vi "Host - 2954 - 6592R Rx Streaming.vi"() -> ()   [LabVIEW 2018, in "Stream-2954-6592R.lvlib"]
uses:
  Stream-2954-6592R.lvlib
  <vilib>/userDefined/Silver/nirio_resource_slv.ctl
  TypeDefs/USRP Configuration.ctl
  TypeDefs/Rx Config.ctl
  2954/SubVIs/Start Trigger.ctl
  TDMS Raw to Channels/Previewed Channel - Enum.ctl
  <instrlib>/niUsrpRio/Config/v1/Host/Public/niUsrpRio Session.ctl
  <instrlib>/_niInstr/Register Bus/v0/Host/Public/Register Bus Session.ctl
  <instrlib>/_niInstr/Register Bus/v0/Host/Private/Session Data.ctl
  <instrlib>/niUsrpRio/Config/v1/Host/Private/DB Queue Reference.ctl
  <instrlib>/niUsrpRio/Config/v1/Host/Private/Daughterboard Data.ctl
  <instrlib>/niUsrpRio/Config/v1/Host/Private/ATR state data.ctl
  <instrlib>/niUsrpRio/Config/v1/Host/Private/Antenna Configuration.ctl
  <instrlib>/niUsrpRio/Config/v1/Host/Private/CPLD Power Mode.ctl
  <instrlib>/niUsrpRio/Config/v1/Host/Public/EEPROM Header.ctl
  <instrlib>/niUsrpRio/Config/v1/Host/Public/EEPROM Device Data Header.ctl
  <instrlib>/niUsrpRio/Config/v1/Host/Public/EEPROM Characterization Header.ctl
  <instrlib>/niUsrpRio/Config/v1/Host/Public/Characterization Data.ctl
  <instrlib>/niUsrpRio/Config/v1/Host/Public/IQ Imbalance.ctl
  TypeDefs/States.ctl
  <vilib>/FPGAPlugInAG/Dynamic/niLvFpga_Close_Dynamic.vi
  <vilib>/rvi/interface/nirviCloseFPGA/nirviCloseFPGA.xnode
  <instrlib>/_niInstr/Register Bus/v0/Host/niInstr Register Bus v0 Host.lvlib
  <instrlib>/niUsrpRio/Config/v1/Host/niUsrpRio Config v1 Host.lvlib
panel:
  in  "Previewed Channel":T1=enum."RF1"
  in  "Rx config":T2={"rf enable 0"=TRUE, "rf config 0"={"antenna"="RX2", "frequency"=2000000000.0, "lo frequency"=-1.0, "level"=0.0}, "rf enable 1"=TRUE, "rf config 1"={"antenna"="RX2", "frequency"=2000000000.0, "lo frequency"=-1.0, "level"=0.0}, "transfer mode"=enum."Continuous", "sample rate"=200000000.0, "start trigger"=enum."Software"} {"sample rate" format="%#.3pS/s"; "rf config 1"."level" format="%#_gdBm"; "rf config 1"."lo frequency" format="%#.3pHz"; "rf config 1"."frequency" format="%#.3pHz"; "rf config 0"."level" format="%#_gdBm"; "rf config 0"."lo frequency" format="%#.3pHz"; "rf config 0"."frequency" format="%#.3pHz"}
  in  "USRP Configuration":T4={"USRP RIO Resources"=["USRP-2954_160MHz"], "reference frequency source"="Internal"}
  in  "Exit":bool
  in  "Stop":bool
  in  "Run":bool
  out "Throughput (B/s)":dbl[](array[numeric])=[800000000.0, 800000000.0] format="%#.3p"
  out "Power Spectral Density (PSD)":cluster{"f0":dbl, "df":dbl, "magnitude":dbl[]}(graph)
  in  "File Path: (path\\desired  name | all channels are named automatically)":path=path "R:/USRP_recording"
  in  "6592R Resources":T5[](array[typedef])=["HSS"]
  # "Rx Aurora - 2 Channel Record Demo"
  # "Hardware Settings"
  # "Recording Settings"
  # "Throughput (B/s)"
  # "Channel Preview"
  # "Control Demo"
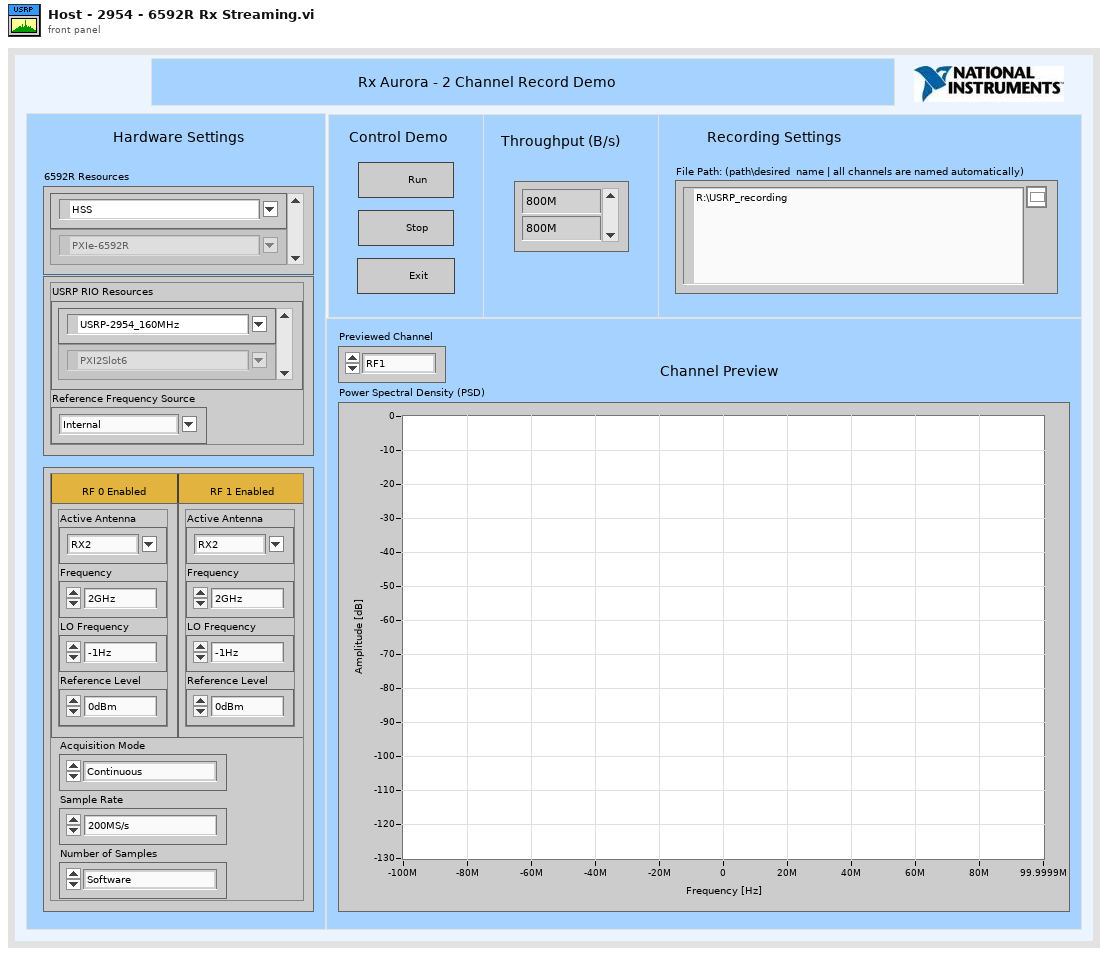
[diagram p1: front panel]
types:
  T1 = typedef "Previewed Channel - Enum.ctl" = enum16{"RF0", "RF1"}
  T2 = typedef "Rx Config.ctl" = cluster{"rf enable 0":bool, "rf config 0":cluster{"antenna":string, "frequency":dbl, "lo frequency":dbl, "level":dbl}, "rf enable 1":bool, "rf config 1":cluster{"antenna":string, "frequency":dbl, "lo frequency":dbl, "level":dbl}, "transfer mode":enum16{"Finite", "Continuous"}, "sample rate":dbl, "start trigger":T3}
  T3 = typedef "Start Trigger.ctl" = enum8{"Software", "Digital Edge", "Rx Start Trigger", "Tx Start Trigger", "Immediate", "Future Time Event"}
  T4 = typedef "USRP Configuration.ctl" = cluster{"USRP RIO Resources":T5[], "reference frequency source":string}
  T5 = typedef "nirio_resource_slv.ctl" = tag
  T6 = typedef "niUsrpRio Config v1 Host.lvlib/niUsrpRio Session.ctl" = cluster{"FPGA Interface":refnum<k20>, "RIO Interface Number":u32, "Data Clock Rate":u32, "FPGA Data Clock Rate":u32, "Global Settings Register Bus":T7, "Radio 0 Settings Register Bus":T7, "Radio 1 Settings Register Bus":T7, "Radio Settings Bus Semaphore":T8, "DB Queues":T9[], "Characterization Data Valid?":bool, "EEPROM Header":T10, "Device Data Header":T11, "EEPROM Characterization Header":T12, "Characterization Data":T13[], "FPGA Current Version":u32, "FPGA Oldest Compatible Version":u32, "Fixed Logic Current Version":u32, "Fixed Logic Oldest Compatible Version":u32, "FPGA Radio Settings Bus Current Version":u32, "FPGA Radio Settings Bus Oldest Compatible Version":u32, "FPGA Board Config Current Version":u32, "FPGA Board Config Oldest Compatible Version":u32, "Daughterboard Clock Rate":u32, "daughterboard configuration session handles":u64[]}
  T7 = typedef "niInstr Register Bus v0 Host.lvlib/Register Bus Session.ctl" = refnum<queue>
  T8 = typedef "Semaphore RefNum" = refnum<k1>
  T9 = typedef "niUsrpRio Config v1 Host.lvlib/DB Queue Reference.ctl" = refnum<queue>
  T10 = typedef "niUsrpRio Config v1 Host.lvlib/EEPROM Header.ctl" = cluster{"Checksum":u32, "Product Code":u16, "Hardware Current Version":u16, "Hardware Oldest Compatible Version":u16, "EEPROM Map Current Version":u16, "EEPROM Map Oldest Compatible Version":u16, "User Password":string, "Pointer to Factory Header":u32, "Pointer to User Header":u32, "Recommended Interval":u16, "Number of Reserved Bytes":i32, "Number of Daughterboards":u8, "Daughterboard IDs":u16[], "Daughterboard Serial Numbers":string[]}
  T11 = typedef "niUsrpRio Config v1 Host.lvlib/EEPROM Device Data Header.ctl" = cluster{"Checksum":u32, "Number of Channels":u8, "Number of Gain Settings":u16[], "Pointer to Characterization Data":u32[], "Number of Reserved Bytes":i32, "Number of Frequencies":u16[]}
  T12 = typedef "niUsrpRio Config v1 Host.lvlib/EEPROM Characterization Header.ctl" = cluster{"Checksum":u32, "Date":timestamp, "Temperature":sgl, "Misc. Info":string, "Pointer to Device Data Header":u32, "Number of Reserved Bytes":i32}
  T13 = typedef "niUsrpRio Config v1 Host.lvlib/Characterization Data.ctl" = cluster{"Gains[dB]":dbl[], "Frequencies [Hz]":dbl[], "IQ Imbalance Table":T14[], "Measured Gains[dB]":dbl[][]}
  T14 = typedef "niUsrpRio Config v1 Host.lvlib/IQ Imbalance.ctl" = cluster{"Gain Imbalance [linear]":dbl, "Phase Imbalance [radians]":dbl, "Offset":cdb}
  T15 = cluster{"HS-Serial Resource":T5[], "USRP Configuration":T4, "File Path":path, "Refnum out":refnum<k20>[], "2 Ports?":bool[], "niUsrpRio Session":T6[], "Simulate Data?":bool, "TDMS Refnums out":refnum<k34>[], "rx config":T2}
  T16 = typedef "States.ctl" = enum16{"Choose Settings", "Exit", "Configure", "Run", "Close", "Shutdown", "transition to Run"}
  T17 = enum8{"Enabled", "Disabled", "Disabled and Grayed Out"}
  T18 = typedef "Rx Channels.ctl" = cluster{"rx config":cluster{"channel configuration":cluster{"channel enable":bool, "channel configuration":cluster{"antenna":string, "frequency":dbl, "lo frequency":dbl, "level":dbl}}[], "transfer mode":enum16{"Finite", "Continuous"}, "sample rate":dbl, "number of samples":u32, "start trigger":T3}, "reference frequency source":string, "rx.data sink":enum16{"SFP Port 0", "SFP Port 1", "Host"}, "rx.enabled channels":string[], "vertical range":dbl[], "rx.coerced configurations":cluster{"coerced frequencies":dbl[], "coerced lo frequencies":dbl[], "coerced levels":dbl[], "coerced sample rates":dbl[]}}
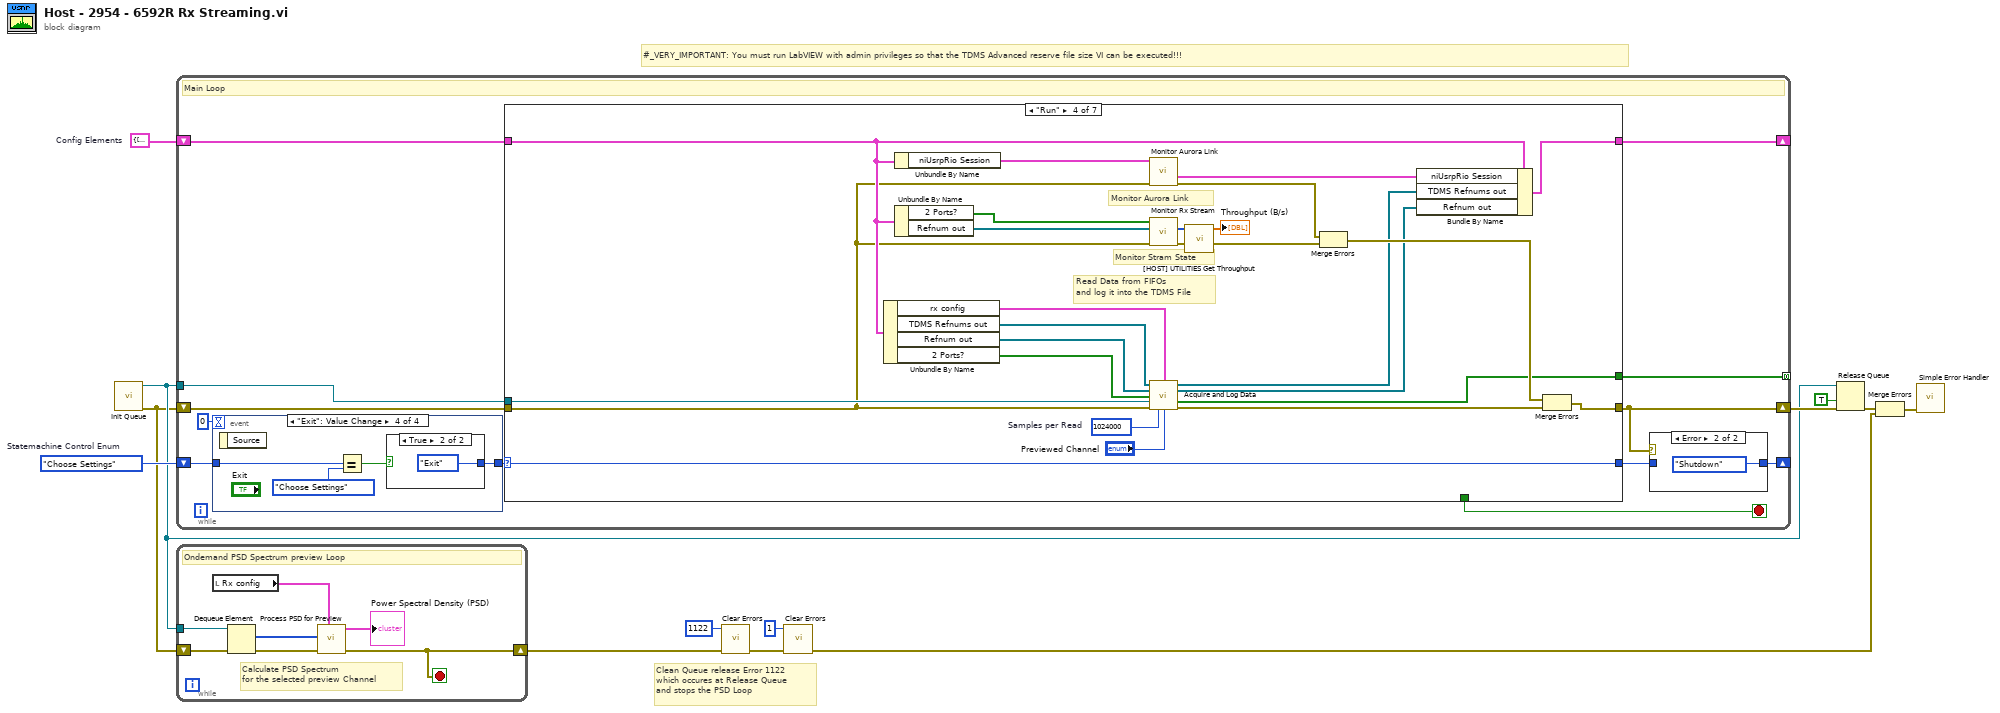
[diagram p0: block diagram]
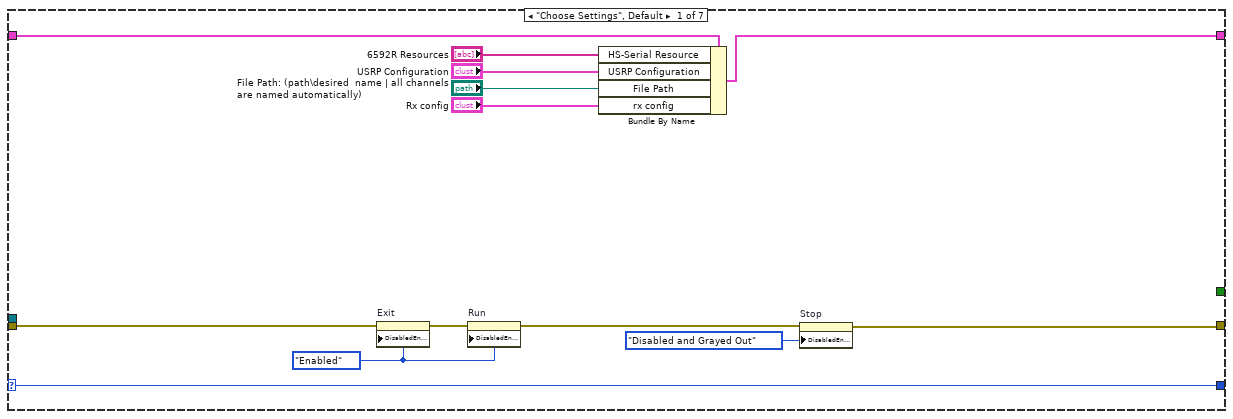
[diagram p3: hidden frame]
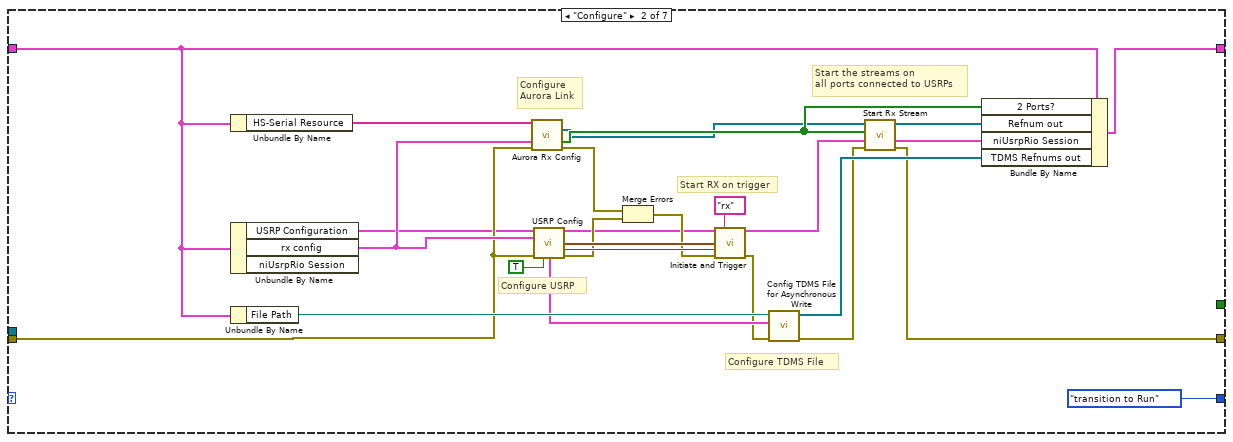
[diagram p4: hidden frame]
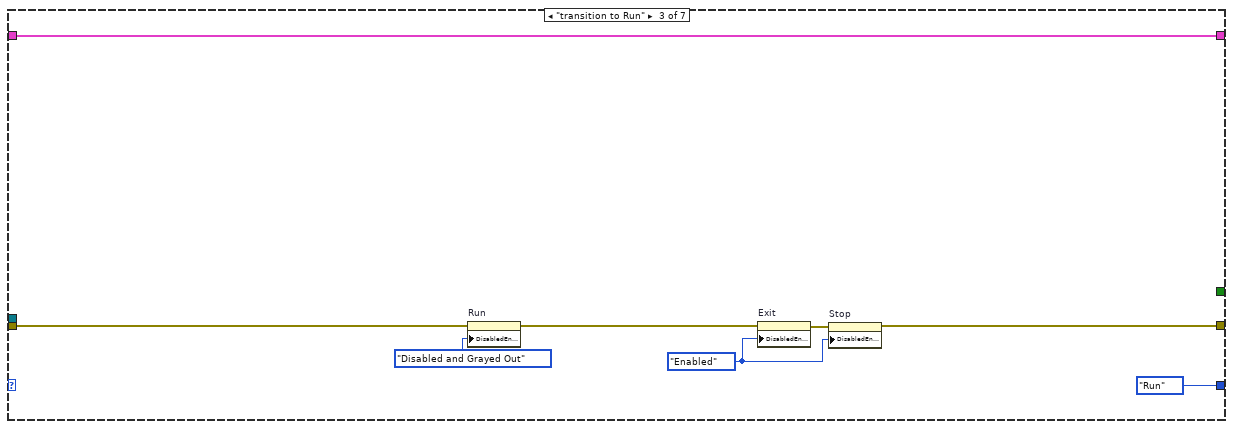
[diagram p5: hidden frame]
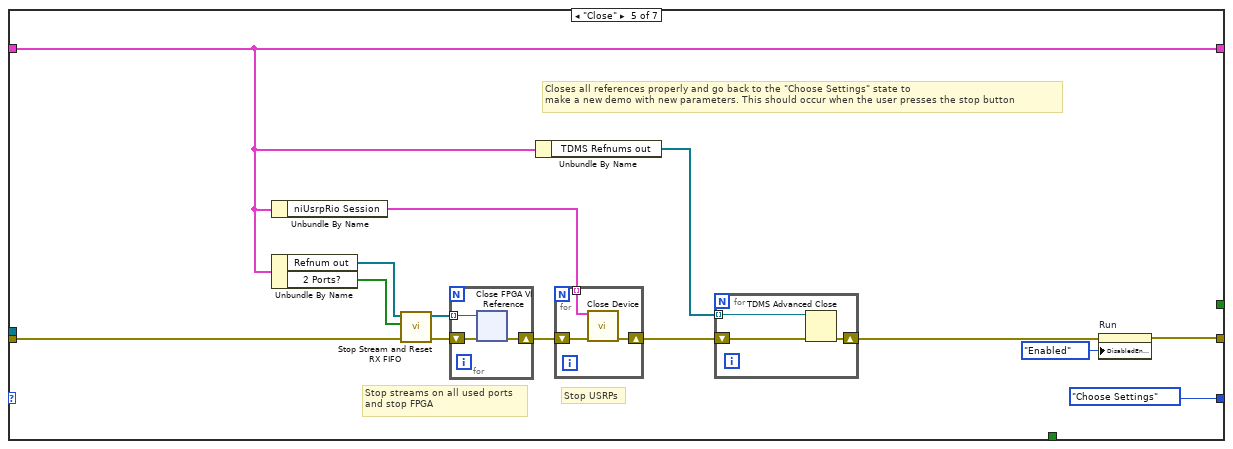
[diagram p6: hidden frame]
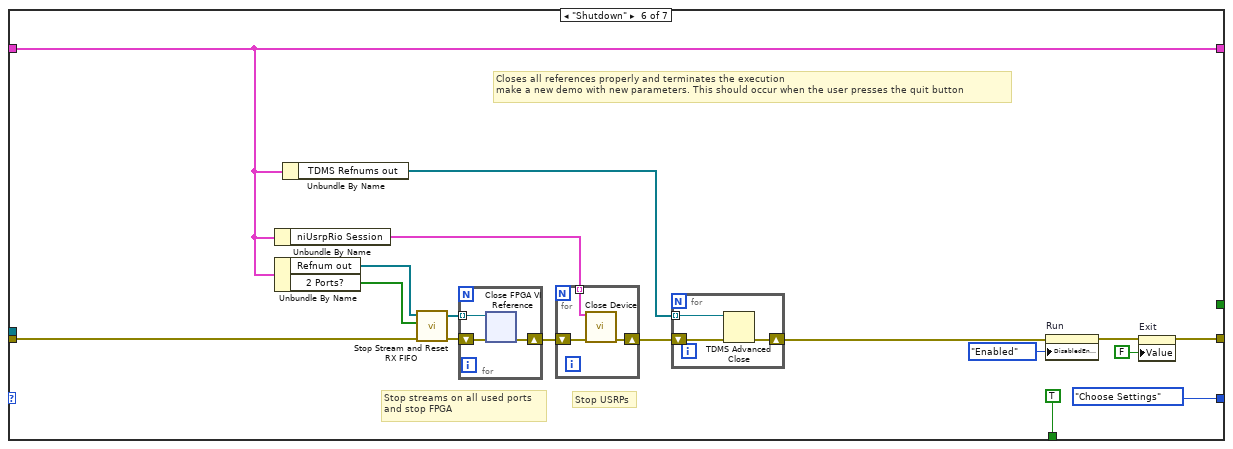
[diagram p7: hidden frame]
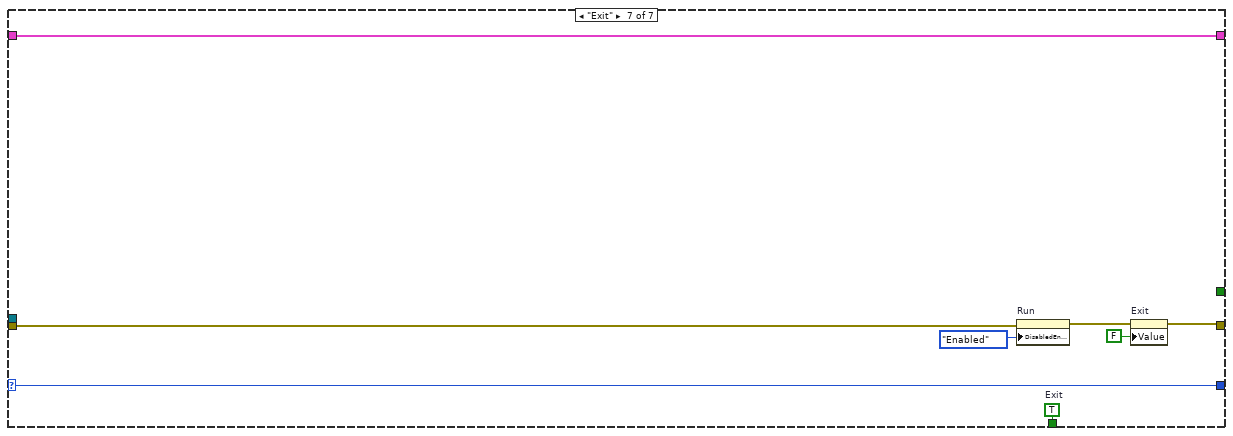
[diagram p8: hidden frame]
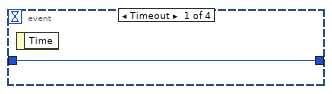
[diagram p9: hidden frame]
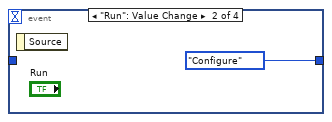
[diagram p10: hidden frame]
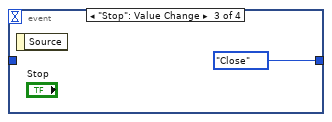
[diagram p11: hidden frame]
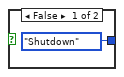
[diagram p12: hidden frame]
diagram:
  w4 = T15 {"HS-Serial Resource"=[], "USRP Configuration"={"USRP RIO Resources"=["USRP-2945"], "reference frequency source"="Internal"}, "File Path"=path "", "Refnum out"=[], "2 Ports?"=[], "niUsrpRio Session"=[], "Simulate Data?"=FALSE, "TDMS Refnums out"=[], "rx config"={"rf enable 0"=TRUE, "rf config 0"={"antenna"="RX2", "frequency"=2000000000.0, "lo frequency"=-1.0, "level"=0.0}, "rf enable 1"=TRUE, "rf config 1"={"antenna"="RX2", "frequency"=2000000000.0, "lo frequency"=-1.0, "level"=0.0}, "transfer mode"=enum."Finite", "sample rate"=10000000.0, "start trigger"=enum."Immediate"}}  # Config Elements
  w13 = States."Choose Settings"  # Statemachine Control Enum
  # "Clean Queue release Error 1122\nwhich occures at Release Queue \nand stops the PSD Loop"
  # "#_VERY_IMPORTANT: You must run LabVIEW with admin privileges so that the TDMS Advanced reserve file size VI can be executed!!!"
  n1 = call "Init Queue.vi"() -> ("error out"=w6:errorcluster, "Queue out"=w7:refnum<queue>)  [unwired: 10 in]
  n2 = while {
    shift-right: [w19] -> _
    shift-left: w13 -> [w25]
    shift-right: [w18] -> w12
    shift-left: w6 -> [w22]
    shift-right: [w16] -> _
    shift-left: w4 -> [w17]
    tunnel: w7 -> [w15]
    tunnel: [w14] -> _ mode=concatenating
    stop <- w21 stop-if-true
    # "Main Loop"
    n3 = event shown="[3] \"Exit\": Value Change" {
      selector: _ -> [_ _ _ _]
      dyn-events: _ -> [_ _ _ _]
      timeout: 0 -> [_ _ _ _]
      tunnel: [w156 States."Configure" States."Close" w160] -> w24
      tunnel: w25 -> [w156 _ _ w161]
      event Timeout {
        n4 = event-data() -> ()  [unwired: 1 in, 1 out]
      }
      event "Run": Value Change {
        n5 = event-data() -> ()  [unwired: 1 in, 1 out]
      }
      event "Stop": Value Change {
        n6 = event-data() -> ()  [unwired: 1 in, 1 out]
      }
      event "Exit": Value Change {
        n7 = event-data() -> ()  [unwired: 1 in, 1 out]
        n8 = Equal?(x=w161, y=States."Choose Settings") -> (x = y?=w159:bool)
        n9 = case shown="True" w159 {
          tunnel: [States."Shutdown" States."Exit"] -> w160
          frame False {
          }
          frame True {
          }
        }
      }
    }
    n10 = case shown="\"Run\"" w24 {
      selector: w24 -> [w31 _ _ w96 _ _ w148]
      tunnel: [w30 w55 w72 w93 w104 w128 w152] -> w18
      tunnel: [w31 States."transition to Run" States."Run" w96 States."Choose Settings" States."Choose Settings" w148] -> w20
      tunnel: w22 -> [w36 w43 w69 w85 w99 w122 w149]
      tunnel: [_ _ _ _ _ TRUE w154] -> w21
      tunnel: w17 -> [w40 w61 w71 w94 w106 w132 w155]
      tunnel: [w37 w60 w71 w92 w106 w132 w155] -> w16
      tunnel: w15 -> [_ _ _ w86 _ _ _]
      tunnel: [_ _ _ w79 _ _ _] -> w14
      frame "Choose Settings", Default {
        w35 = T17."Enabled" ("Disabled")
        n11 = property on="Exit" class="Bool (strict)"(error in=w36, "DisabledEnum"=w35) -> (error out=w34:errorcluster)  [unwired: 1 in, 1 out]
        n12 = property on="Run" class="Bool"(error in=w34, "DisabledEnum"=w35) -> (error out=w33:errorcluster)  [unwired: 1 in, 1 out]
        n13 = Bundle By Name(cluster=w40, "HS-Serial Resource"="6592R Resources", "USRP Configuration"="USRP Configuration", "File Path"="File Path: (path\\desired  name | all channels are named automatically)", "rx config"="Rx config") -> (w37:T15)
        n14 = property on="Stop" class="Bool"(error in=w33, "DisabledEnum"=T17."Disabled and Grayed Out" ("Disabled")) -> (error out=w30:errorcluster)  [unwired: 1 in, 1 out]
      }
      frame "Configure" {
        # "Start RX on trigger"
        # "Configure TDMS File"
        # "Start the streams on \nall ports connected to USRPs"
        # "Configure \nAurora Link"
        # "Configure USRP"
        n15 = Unbundle By Name(w61) -> ("HS-Serial Resource"=w45:T5[])
        n16 = Unbundle By Name(w61) -> ("USRP Configuration"=w41:T4, "rx config"=w44:T2)  [unwired: 1 out]
        n17 = Unbundle By Name(w61) -> ("File Path"=w59:path)
        n18 = call "Aurora Rx Config.vi"("6592R Resources"=w45, "rx config"=w44, "error in (no error)"=w43) -> ("Refnum out"=w46:refnum<k20>[], "2 Ports?"=w47:bool[], "error out"=w48:errorcluster)  [unwired: 8 in, 2 out]
        n19 = call "USRP Config.vi"("USRP Configuration"=w41, "rx config"=w44, "error in (no error)"=w43, "Rx?"=TRUE) -> ("niUsrpRio Session"=w50:T6[], "start trigger out"=w64:T3, "Time Stamp"=w63:timestamp, "rx channels"=w57:T18, "error out"=w52:errorcluster)  [unwired: 3 in, 4 out]
        n20 = Merge Errors(w48, w52) -> (w53:errorcluster)
        n21 = call "Initiate and Trigger.vi"("niUsrpRio Sessions"=w50, "scope"="rx", "start trigger"=w64, "start trigger time"=w63, "error in"=w53) -> ("niUsrpRio Sessions (out)"=w54:T6[], "error out"=w56:errorcluster)  [unwired: 9 in]
        n22 = call "Config TDMS File for Asynchronous Write.vi"("error in (no error)"=w56, "rx channels"=w57, "base path"=w59) -> ("error out"=w51:errorcluster, "Refnums out"=w58:refnum<k34>[])  [unwired: 7 in]
        n23 = call "Start Rx Stream.vi"("error in (no error)"=w51, "2 Ports?"=w47, "Refnum in"=w46) -> ("error out"=w55:errorcluster, "Refnum out"=w49:refnum<k20>[])  [unwired: 7 in]
        n24 = Bundle By Name(cluster=w61, "2 Ports?"=w47, "Refnum out"=w49, "niUsrpRio Session"=w54, "TDMS Refnums out"=w58) -> (w60:T15)
      }
      frame "transition to Run" {
        w70 = T17."Enabled" ("Disabled")
        n25 = property on="Run" class="Bool"(error in=w69, "DisabledEnum"=T17."Disabled and Grayed Out" ("Disabled")) -> (error out=w68:errorcluster)  [unwired: 1 in, 1 out]
        n26 = property on="Exit" class="Bool (strict)"(error in=w68, "DisabledEnum"=w70) -> (error out=w73:errorcluster)  [unwired: 1 in, 1 out]
        n27 = property on="Stop" class="Bool"(error in=w73, "DisabledEnum"=w70) -> (error out=w72:errorcluster)  [unwired: 1 in, 1 out]
      }
      frame "Run" {
        w82 = u32 1024000  # Samples per Read
        # "Read Data from FIFOs \nand log it into the TDMS File"
        # "Monitor Stram State"
        # "Monitor Aurora Link"
        n28 = Unbundle By Name(w94) -> ("rx config"=w75:T2, "TDMS Refnums out"=w84:refnum<k34>[], "Refnum out"=w88:refnum<k20>[], "2 Ports?"=w87:bool[])
        n29 = Unbundle By Name(w94) -> ("niUsrpRio Session"=w81:T6[])
        n30 = Unbundle By Name(w94) -> ("2 Ports?"=w95:bool[], "Refnum out"=w78:refnum<k20>[])
        n31 = call "Monitor Aurora Link.vi"("error in (no error)"=w85, "niUsrpRio Sessions (In)"=w81) -> ("error out"=w91:errorcluster, "niUsrpRio Sessions (Out)"=w76:T6[])  [unwired: 5 in, 3 out]
        n32 = call "Monitor Rx Stream.vi"("error in (no error)"=w85, "Refnum in"=w78, "2 Ports?"=w95) -> ("error out"=w77:errorcluster, "Samples Transferred"=w97:u64[])  [unwired: 6 in, 1 out]
        n33 = call "Acquire and Log Data.vi"("TDMS Refnums in"=w84, "rx config"=w75, "Refnum in"=w88, "2 USRPs?"=w87, "Data Queue in"=w86, "error in (no error)"=w85, "Samples per Read"=w82, "Previewed Channel"="Previewed Channel") -> ("TDMS Refnums out"=w83:refnum<k34>[], "Refnum out"=w89:refnum<k20>[], "Array"=w79:bool[], "error out"=w80:errorcluster)  [unwired: 4 in]
        n34 = call "[HOST] UTILITIES Get Throughput.vi"("Samples"=w97) -> ("Throughput"=→"Throughput (B/s)":dbl[])  [unwired: 10 in]
        n35 = Merge Errors(w91, w77) -> (w90:errorcluster)
        n36 = Bundle By Name(cluster=w94, "niUsrpRio Session"=w76, "TDMS Refnums out"=w83, "Refnum out"=w89) -> (w92:T15)
        n37 = Merge Errors(w90, w80) -> (w93:errorcluster)
      }
      frame "Close" {
        # "Closes all references properly and go back to the \"Choose Settings\" state to \nmake a new demo with new parameters. This should occur when the user presses the stop button"
        # "Stop streams on all used ports \nand stop FPGA"
        # "Stop USRPs"
        n38 = Unbundle By Name(w106) -> ("niUsrpRio Session"=w107:T6[])
        n39 = Unbundle By Name(w106) -> ("Refnum out"=w100:refnum<k20>[], "2 Ports?"=w108:bool[])
        n40 = call "Stop Stream and Reset RX FIFO.vi"("error in (no error)"=w99, "2 USRPs?"=w108, "Refnum in"=w100) -> ("error out"=w111:errorcluster, "Refnum out"=w112:refnum<k20>[])  [unwired: 7 in]
        n41 = for {
          tunnel: w112 -> [w120] mode=indexing
          shift-right: [w121] -> w110
          shift-left: w111 -> [w119]
          n42 = xnode "Close FPGA VI Reference"("FPGA VI Reference In"=w120, "error in"=w119) -> ("error out"=w121:errorcluster)
        }
        n43 = Unbundle By Name(w106) -> ("TDMS Refnums out"=w103:refnum<k34>[])
        n44 = for {
          shift-right: [w117] -> w102
          shift-left: w110 -> [w118]
          tunnel: w107 -> [w116] mode=indexing
          n45 = call "Close Device.vi"("niUsrpRio Session"=w116, "error in"=w118) -> ("error out"=w117:errorcluster)  [unwired: 13 in]
        }
        n46 = for {
          shift-right: [w114] -> w101
          shift-left: w102 -> [w115]
          tunnel: w103 -> [w113] mode=indexing
          n47 = TDMS Advanced Close(8:w115, 11:w113) -> (0:w114:errorcluster)  [unwired: 2 in, 1 out]
        }
        n48 = property on="Run" class="Bool"(error in=w101, "DisabledEnum"=T17."Enabled" ("Disabled")) -> (error out=w104:errorcluster)  [unwired: 1 in, 1 out]
      }
      frame "Shutdown" {
        # "Stop streams on all used ports \nand stop FPGA"
        # "Closes all references properly and terminates the execution\nmake a new demo with new parameters. This should occur when the user presses the quit button"
        # "Stop USRPs"
        n49 = Unbundle By Name(w132) -> ("niUsrpRio Session"=w133:T6[])
        n50 = Unbundle By Name(w132) -> ("Refnum out"=w123:refnum<k20>[], "2 Ports?"=w134:bool[])
        n51 = Unbundle By Name(w132) -> ("TDMS Refnums out"=w126:refnum<k34>[])
        n52 = call "Stop Stream and Reset RX FIFO.vi"("error in (no error)"=w122, "2 USRPs?"=w134, "Refnum in"=w123) -> ("error out"=w137:errorcluster, "Refnum out"=w138:refnum<k20>[])  [unwired: 7 in]
        n53 = for {
          tunnel: w138 -> [w146] mode=indexing
          shift-right: [w147] -> w136
          shift-left: w137 -> [w145]
          n54 = xnode "Close FPGA VI Reference"("FPGA VI Reference In"=w146, "error in"=w145) -> ("error out"=w147:errorcluster)
        }
        n55 = for {
          shift-right: [w143] -> w125
          shift-left: w136 -> [w144]
          tunnel: w133 -> [w142] mode=indexing
          n56 = call "Close Device.vi"("niUsrpRio Session"=w142, "error in"=w144) -> ("error out"=w143:errorcluster)  [unwired: 13 in]
        }
        n57 = for {
          shift-right: [w140] -> w124
          shift-left: w125 -> [w141]
          tunnel: w126 -> [w139] mode=indexing
          n58 = TDMS Advanced Close(8:w141, 11:w139) -> (0:w140:errorcluster)  [unwired: 2 in, 1 out]
        }
        n59 = property on="Run" class="Bool"(error in=w124, "DisabledEnum"=T17."Enabled" ("Disabled")) -> (error out=w127:errorcluster)  [unwired: 1 in, 1 out]
        n60 = property on="Exit" class="Bool (strict)"(error in=w127, "Value"=FALSE ("Exit")) -> (error out=w128:errorcluster)  [unwired: 1 in, 1 out]
      }
      frame "Exit" {
        w154 = TRUE  # Exit
        n61 = property on="Run" class="Bool"(error in=w149, "DisabledEnum"=T17."Enabled" ("Disabled")) -> (error out=w150:errorcluster)  [unwired: 1 in, 1 out]
        n62 = property on="Exit" class="Bool (strict)"(error in=w150, "Value"=FALSE ("Exit")) -> (error out=w152:errorcluster)  [unwired: 1 in, 1 out]
      }
    }
    n63 = case shown="Error" w18 {
      tunnel: [w26 States."Shutdown"] -> w19
      tunnel: w20 -> [w26 _]
      frame No Error {
      }
      frame Error {
      }
    }
  }
  n64 = while {
    shift-right: [w166] -> w8
    shift-left: w6 -> [w171]
    tunnel: w7 -> [w169]
    stop <- w166 stop-if-true
    # "Calculate PSD Spectrum\nfor the selected preview Channel"
    # "Ondemand PSD Spectrum preview Loop"
    n65 = local read "Rx config"() -> (w165:T2)
    n66 = Dequeue Element(queue=w169, error in (no error)=w171) -> (element=w167:u64[], error out=w170:errorcluster)  [unwired: 1 in, 2 out]
    n67 = call "Process PSD for Preview.vi"("Rx config"=w165, "error in (no error)"=w170, "Data Array"=w167) -> ("error out"=w166:errorcluster, "Power Spectrum / PSD"=→"Power Spectral Density (PSD)":cluster{"f0":dbl, "df":dbl, "magnitude":dbl[]})  [unwired: 7 in]
  }
  n68 = call <vilib>:"Clear Errors.vi"("error in (no error)"=w8, "specific error code to clear (0: all)"=1122) -> ("error out"=w3:errorcluster)  [unwired: 4 in, 1 out]
  n69 = call <vilib>:"Clear Errors.vi"("error in (no error)"=w3, "specific error code to clear (0: all)"=1) -> ("error out"=w2:errorcluster)  [unwired: 4 in, 1 out]
  n70 = Release Queue(queue=w7, force destroy? (F)=TRUE, error in (no error)=w12) -> (error out=w10:errorcluster)  [unwired: 2 out]
  n71 = Merge Errors(w10, w2) -> (w9:errorcluster)
  n72 = call <vilib>:"Simple Error Handler.vi"("error in (no error)"=w9) -> ()  [unwired: 4 in, 5 out]
